vi "Teleop.vi"(10 "Match Info":T1={"Autonomous Elapsed Seconds"=0.0, "TeleOp Elapsed Seconds"=0.0, "Disabled Elapsed Seconds"=0.0, "Visited Autonomous"=FALSE, "Visited TeleOp"=FALSE, "Visited Disabled"=FALSE, "Autonomous Settings"={"Autonomous Style"=enum."Independent", "VI Refnum"=refnum}}, 11 "Call Context":T2) -> ()   [LabVIEW 2013]
doc: "This VI is called for each TeleOp packet received from the DS where the robot is not disabled. It is often used to read from the joysticks and update I/O or to update setpoints for timed control loops. It should complete and return within 20 milliseconds or it may miss DS packets."
uses:
  <vilib>/Rock Robotics/WPI/DriverStation/WPI_DriverStationDerivedRobotMode.ctl
  <vilib>/Rock Robotics/WPI/DriverStation/WPI_DriverStationMatch Info.ctl
  KariQueue/TeleopInstruction.ctl
  Robot Global Data.vi
  <vilib>/Rock Robotics/WPI/Joystick/WPI_JoystickGetSetRefNum.vi
panel:
  out "TeleopTime":u32
  in  "error in (no error)":errorcluster
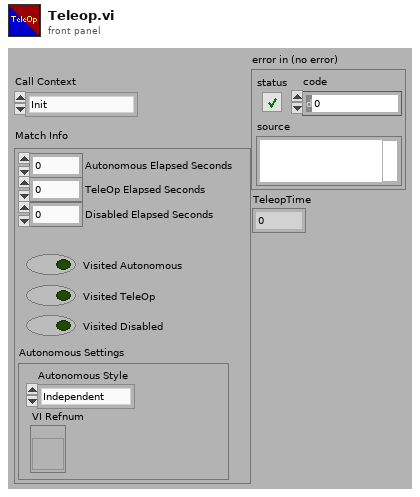
[diagram p1: front panel]
types:
  T1 = typedef "WPI_DriverStationMatch Info.ctl" = cluster{"Autonomous Elapsed Seconds":dbl, "TeleOp Elapsed Seconds":dbl, "Disabled Elapsed Seconds":dbl, "Visited Autonomous":bool, "Visited TeleOp":bool, "Visited Disabled":bool, "Autonomous Settings":cluster{"Autonomous Style":enum16{"Iterative", "Independent"}, "VI Refnum":refnum<vi>}}
  T2 = typedef "WPI_DriverStationDerivedRobotMode.ctl" = enum16{"Init", "Execute", "Stop"}
  T3 = typedef "WPI_JoystickDevRef.ctl" = cluster{"Device":T4}
  T4 = typedef "WPI_JoystickDeviceEnum.ctl" = enum16{"USB 1", "USB 2", "USB 3", "USB 4", "Kinect 1", "Kinect 2"}
  T5 = typedef "WPI_JoystickButtonState.ctl" = cluster{"Button 1":bool, "Button 2":bool, "Button 3":bool, "Button 4":bool, "Button 5":bool, "Button 6":bool, "Button 7":bool, "Button 8":bool, "Button 9":bool, "Button 10":bool, "Button 11":bool, "Button 12":bool}
  T6 = cluster{"axis 1 (x)":dbl, "axis 2 (y)":dbl, "axis 3 (throttle)":dbl, "axis 4":dbl, "axis 5":dbl, "axis 6":dbl}
  T7 = typedef "TeleopInstruction.ctl" = cluster{"cDriveLeft":dbl, "cDriveRight":dbl, "cHalfDrive":bool, "cStraightDrive":bool, "cSonicShifter":bool}
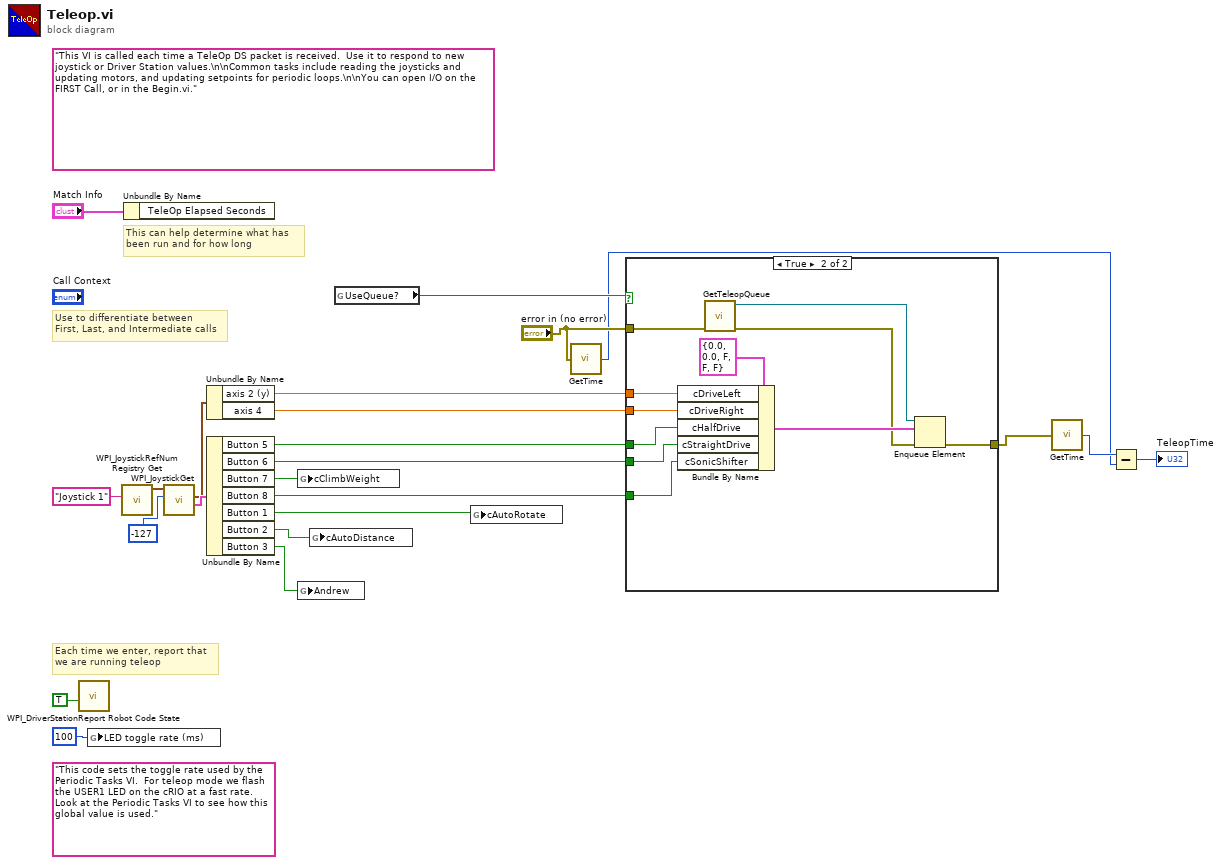
[diagram p0: block diagram]
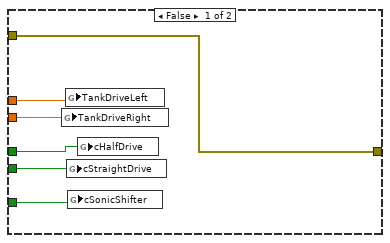
[diagram p2: hidden frame]
diagram:
  (unwired) "This code sets the toggle rate used by the Periodic Tasks VI.  For teleop mode we flash the USER1 LED on the cRIO at a fast rate.  Look at the Periodic Tasks VI to see how this global value is used."
  (unwired) "This VI is called each time a TeleOp DS packet is received.  Use it to respond to new joystick or Driver Station values.\n\nCommon tasks include reading the joysticks and updating motors, and updating setpoints for periodic loops.\n\nYou can open I/O on the FIRST Call, or in the Begin.vi."
  # "Each time we enter, report that\nwe are running teleop"
  # "Use to differentiate between\nFirst, Last, and Intermediate calls"
  # "This can help determine what has\nbeen run and for how long"
  n1 = call <vilib>:"WPI_DriverStationReport Robot Code State.vi"("TeleOp"=TRUE ("Autonomous")) -> ()  [unwired: 10 in, 1 out]
  n2 = global write "Robot Global Data.vi" "LED toggle rate (ms)"(u32 100 ("LED ms toggle rate")) -> ()
  n3 = call <vilib>:"WPI_JoystickRefNum Registry Get.vi"("refnum name"="Joystick 1") -> ("JoystickDevRef"=w21:T3)  [unwired: 1 in, 9 out]
  n4 = Unbundle By Name("Match Info") -> ()  [unwired: 1 out]
  n5 = call <vilib>:"WPI_JoystickGet.vi"("Scaler"=i8 -127, "JoystickDevRef"=w21) -> ("Buttons"=w18:T5, "Axes"=w16:T6)  [unwired: 4 out]
  n6 = Unbundle By Name(w16) -> ("axis 2 (y)"=w12:dbl, "axis 4"=w11:dbl)
  n7 = Unbundle By Name(w18) -> ("Button 5"=w10:bool, "Button 6"=w9:bool, "Button 7"=w17:bool, "Button 8"=w7:bool, "Button 1"=w6:bool, "Button 2"=w15:bool, "Button 3"=w14:bool)
  n8 = global write "Robot Global Data.vi" "cClimbWeight"(w17) -> ()
  n9 = global write "Robot Global Data.vi" "Andrew"(w14) -> ()
  n10 = global write "Robot Global Data.vi" "cAutoDistance"(w15) -> ()
  n11 = global read "Robot Global Data.vi" "UseQueue?"() -> (w8:bool)
  n12 = global write "Robot Global Data.vi" "cAutoRotate"(w6) -> ()
  n13 = call "GetTime.vi"("error in"="error in (no error)") -> ("Time"=w2:u32)
  n14 = case shown="True" w8 {
    tunnel: w12 -> [w25 w36]
    tunnel: w11 -> [w26 w35]
    tunnel: w10 -> [w27 w34]
    tunnel: w9 -> [w28 w33]
    tunnel: w7 -> [w29 w32]
    tunnel: [w24 w31] -> w4
    tunnel: "error in (no error)" -> [w24 w30]
    frame False {
      n15 = global write "Robot Global Data.vi" "TankDriveRight"(w26) -> ()
      n16 = global write "Robot Global Data.vi" "TankDriveLeft"(w25) -> ()
      n17 = global write "Robot Global Data.vi" "cStraightDrive"(w28) -> ()
      n18 = global write "Robot Global Data.vi" "cSonicShifter"(w29) -> ()
      n19 = global write "Robot Global Data.vi" "cHalfDrive"(w27) -> ()
    }
    frame True {
      n20 = Bundle By Name(cluster=T7 {"cDriveLeft"=0.0, "cDriveRight"=0.0, "cHalfDrive"=FALSE, "cStraightDrive"=FALSE, "cSonicShifter"=FALSE} ("TeleopInstruction"), "cDriveLeft"=w36, "cDriveRight"=w35, "cHalfDrive"=w34, "cStraightDrive"=w33, "cSonicShifter"=w32) -> (w38:T7)
      n21 = call "GetTeleopQueue.vi"("error in (no error)"=w30) -> ("error out"=w37:errorcluster, "queue out"=w40:refnum<queue>)  [unwired: 9 in]
      n22 = Enqueue Element(queue=w40, element=w38, error in (no error)=w37) -> (error out=w31:errorcluster)  [unwired: 1 in, 2 out]
    }
  }
  n23 = call "GetTime.vi"("error in"=w4) -> ("Time"=w3:u32)
  n24 = Subtract(x=w3, y=w2) -> (x-y=→"TeleopTime":u32)
